vi "onHttpPut (File).vi"(8 "error in":errorcluster, 10 "httpRequest":refnum<class "httpRequest.lvclass">, 11 "http-method in":refnum<class "HttpClient.Basic.lvclass">) -> (0 "error out":errorcluster, 2 "httpResponse":refnum<class "httpResponse.lvclass">, 3 "http-method out":refnum<class "HttpClient.Basic.lvclass">)   [LabVIEW 2020, in "httpClient.lvlib" / "HttpClient.Basic.lvclass"]
uses:
  HttpClient.Basic.lvclass
  HttpClient.Basic.lvclass/HttpClient.Basic.ctl
  <vilib>/httpClient/LabVIEWHTTPClient.lvlib
  <vilib>/httpClient/PUTBuffer.vi
  httpRequest/httpRequest.lvclass
  httpResponse/httpResponse.lvclass
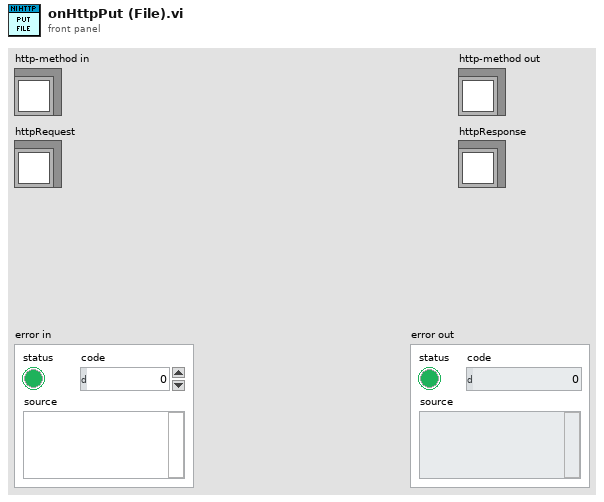
[diagram p1: front panel]
types:
  T1 = typedef "LabVIEWHTTPClient.lvlib/ClientHandle.ctl" = refnum<k1>
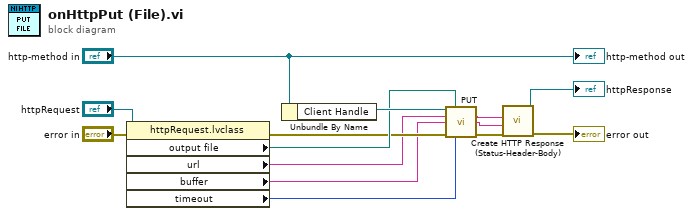
[diagram p0: block diagram]
diagram:
  n1 = property class="httpRequest.lvclass"(reference="httpRequest", error in="error in") -> (error out=w11:errorcluster, "output file"=w12:path, "url"=w8:string, "buffer"=w7:string, "timeout"=w6:i32)  [unwired: 1 out]
  n2 = Unbundle By Name("http-method in") -> ("Client Handle"=w13:T1)
  n3 = call-poly <vilib>:"PUT.vi"("client handle"=w13, "output file"=w12, "url"=w8, "buffer"=w7, "error in (no error)"=w11, "timeout (10000)"=w6) -> ("headers"=w3:string, "body"=w4:string, "error out"=w5:errorcluster)  [unwired: 6 in, 1 out]
  n4 = call "Create HTTP Response (Status-Header-Body).vi"("error in"=w5, "body"=w4, "Headers w/ status line(s)"=w3) -> ("error out"=→"error out":errorcluster, "httpResponse out"=→"httpResponse":refnum<class "httpResponse.lvclass">)  [unwired: 7 in]
  "http-method out" <- "http-method in"
